vi "Lockin.DAQ.Set Initial Value.vi"(8 "error in (no error)":errorcluster, 11 "Lockin.DAQ in":refnum<class "Lockin.DAQ.lvclass">) -> (0 "error out":errorcluster, 3 "Lockin.DAQ out":refnum<class "Lockin.DAQ.lvclass">)   [LabVIEW 2016, in "Lockin.DAQ.lvclass"]
uses:
  Lockin.DAQ.lvclass
  Lockin.DAQ.lvclass/Lockin.DAQ.ctl
  Typedefs/Function-enum.ctl
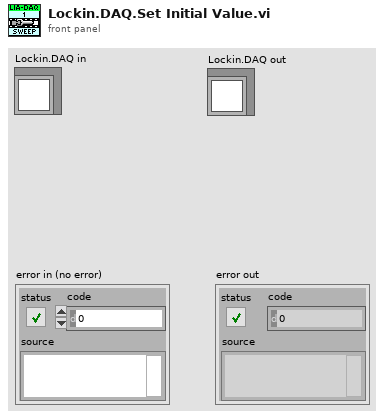
[diagram p1: front panel]
types:
  T1 = typedef "Lockin.DAQ.lvclass/AO-cluster.ctl" = cluster{"Ch":i32[], "Amp (V)":dbl[], "DC (V)":dbl[], "f (Hz)":dbl[], "Phase (°)":dbl[], "Function":T2[], "Sweep?":bool[]}
  T2 = typedef "Lockin.DAQ.lvclass/Function-enum.ctl" = enum16{"Sine", "Triangle", "Square", "Sawtooth"}
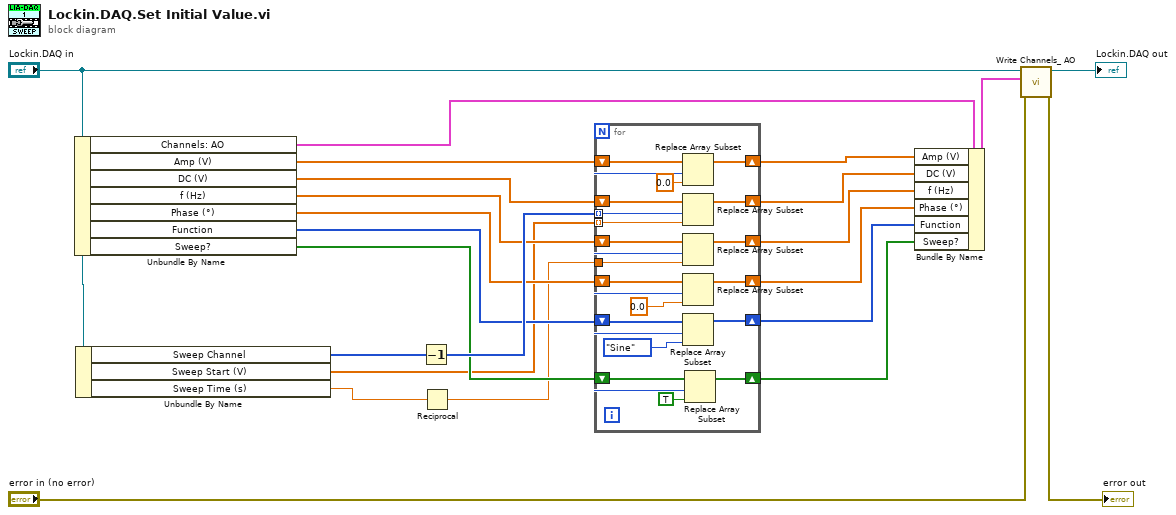
[diagram p0: block diagram]
diagram:
  n1 = Unbundle By Name("Lockin.DAQ in") -> ("Channels: AO"=w3:T1, "Amp (V)"=w18:dbl[], "DC (V)"=w17:dbl[], "f (Hz)"=w16:dbl[], "Phase (°)"=w15:dbl[], "Function"=w14:T2[], "Sweep?"=w13:bool[])
  n2 = Unbundle By Name("Lockin.DAQ in") -> ("Sweep Channel"=w8:i32[], "Sweep Start (V)"=w7:dbl[], "Sweep Time (s)"=w6:dbl)
  n3 = Decrement(x=w8) -> (x-1=w19:i32[])
  n4 = Reciprocal(x=w6) -> (1/x=w5:dbl)
  n5 = for {
    tunnel: w19 -> [w39] mode=indexing
    tunnel: w7 -> [w25] mode=indexing
    tunnel: w5 -> [w24]
    shift-right: [w32] -> w12
    shift-left: w18 -> [w38]
    shift-right: [w31] -> w2
    shift-left: w17 -> [w37]
    shift-right: [w30] -> w11
    shift-left: w16 -> [w36]
    shift-right: [w29] -> w10
    shift-left: w15 -> [w35]
    shift-right: [w28] -> w9
    shift-left: w14 -> [w34]
    shift-right: [w27] -> w1
    shift-left: w13 -> [w33]
    n6 = Replace Array Subset(array=w38, new element=0.0 ("new element/subarray"), index=w39) -> (w32:dbl[])
    n7 = Replace Array Subset(array=w37, new element=w25, index=w39) -> (w31:dbl[])
    n8 = Replace Array Subset(array=w36, new element=w24, index=w39) -> (w30:dbl[])
    n9 = Replace Array Subset(array=w35, new element=0.0 ("new element/subarray"), index=w39) -> (w29:dbl[])
    n10 = Replace Array Subset(array=w34, new element=Function-enum."Sine" ("new element/subarray"), index=w39) -> (w28:T2[])
    n11 = Replace Array Subset(array=w33, new element=TRUE ("new element/subarray"), index=w39) -> (w27:bool[])
  }
  n12 = Bundle By Name(cluster=w3, "Amp (V)"=w12, "DC (V)"=w2, "f (Hz)"=w11, "Phase (°)"=w10, "Function"=w9, "Sweep?"=w1) -> (w20:T1)
  n13 = call "Write Channels_ AO.vi"("error in (no error)"="error in (no error)", "Channels: AO"=w20, "Lockin.DAQ"="Lockin.DAQ in") -> ("error out"=→"error out":errorcluster, "Lockin.DAQ out"=→"Lockin.DAQ out":refnum<class "Lockin.DAQ.lvclass">)  [unwired: 7 in]
